vi "ST_parse_reference_list.vi"(6 "recordset_data":variant[][](array[variant]), 8 "error_in":errorcluster, 11 "command_nmb":u8) -> (0 "error_out":errorcluster, 3 "reference_data_to_PLC":u8[](array[numeric]))   [LabVIEW 2020]
uses:
  ST_reference_info.ctl
  _misc/byte_array_parser/from_STR_to_PLC_STRING[30].vi
  reference_byte_offsset/ref_STRING_offset.vi
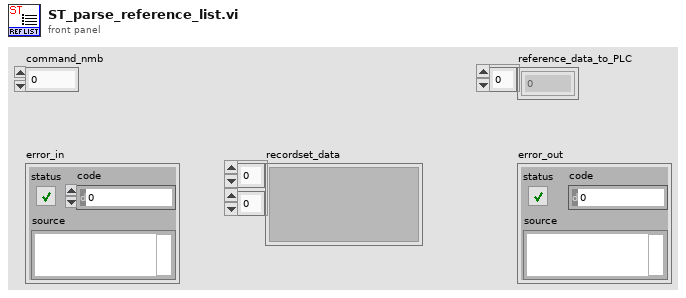
[diagram p1: front panel]
types:
  T1 = typedef "ST_reference_info.ctl" = cluster{"INT_number":i32, "REAL_number":i32, "STRING_number":i32, "STRING_size":i32, "BYTE_array":u8[]}
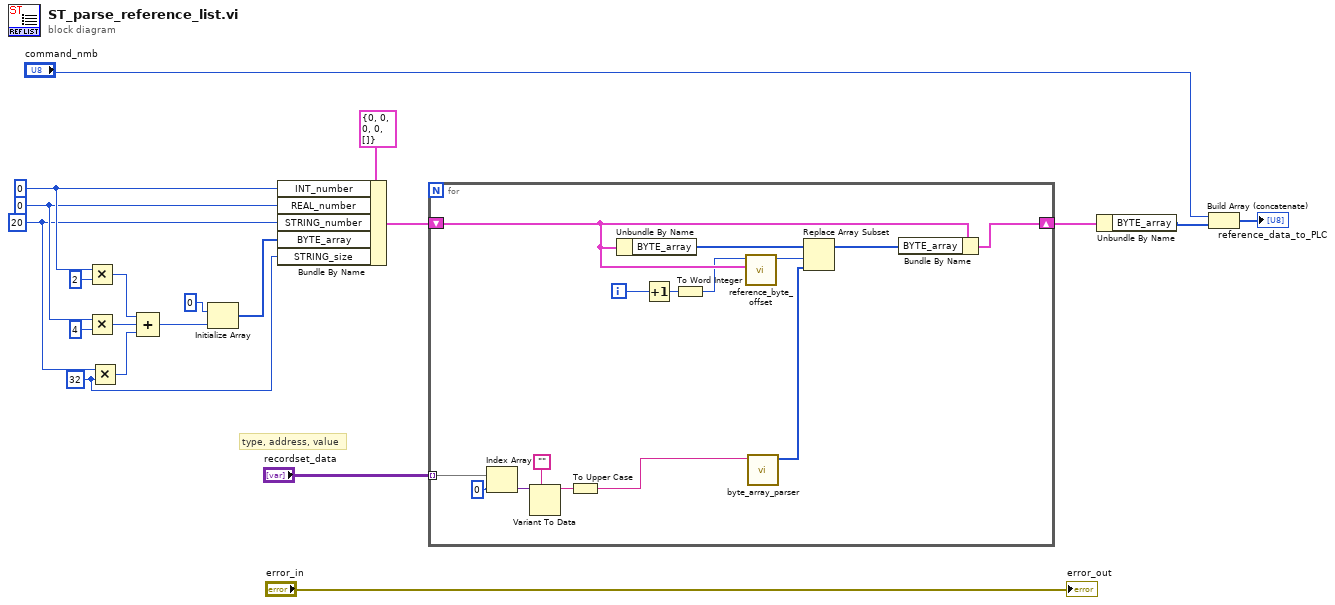
[diagram p0: block diagram]
diagram:
  w4 = 32 ("y")
  w5 = 20 ("STRING_number")
  w6 = 0 ("REAL_number")
  w7 = 0 ("INT_number")
  # "type, address, value"
  n1 = Multiply(x=w7, y=2) -> (x*y=w12:i32)
  n2 = Multiply(x=w6, y=4) -> (x*y=w11:i32)
  n3 = Multiply(x=w5, y=w4) -> (x*y=w10:i32)
  n4 = Compound Arithmetic op=unknown(w12, w11, w10) -> (w9:i32)
  n5 = Initialize Array(u8 0 ("element"), w9) -> (w15:u8[])
  n6 = Bundle By Name(cluster=T1 {"INT_number"=0, "REAL_number"=0, "STRING_number"=0, "STRING_size"=0, "BYTE_array"=[]}, "INT_number"=w7, "REAL_number"=w6, "STRING_number"=w5, "BYTE_array"=w15, "STRING_size"=w4) -> (w17:T1)
  n7 = for {
    tunnel: "recordset_data" -> [w30] mode=indexing
    shift-right: [w29] -> w8
    shift-left: w17 -> [w35]
    i -> [w23]
    n8 = Index Array(array=w30, index=0) -> (element=w33:variant)
    n9 = Variant To Data(type="", Variant=w33) -> (data=w31:string)  [unwired: 1 in, 1 out]
    n10 = To Upper Case(1:w31) -> (0:w24:string)
    n11 = Unbundle By Name(w35) -> ("BYTE_array"=w28:u8[])
    n12 = Increment(x=w23) -> (x+1=w22:i32)
    n13 = To Word Integer(number=w22) -> (16bit integer=w21:i16)
    n14 = call-poly "reference_byte_offset.vi"("ST_reference_info"=w35, "STRING_position"=w21) -> ("reference_byte_array_offset"=w25:i32)  [unwired: 9 in]
    n15 = call-poly "byte_array_parser.vi"("String"=w24) -> ("byte_array"=w26:u8[])  [unwired: 9 in, 1 out]
    n16 = Replace Array Subset(array=w28, new element=w26, index=w25) -> (w27:u8[])
    n17 = Bundle By Name(cluster=w35, "BYTE_array"=w27) -> (w29:T1)
  }
  n18 = Unbundle By Name(w8) -> ("BYTE_array"=w3:u8[])
  n19 = Build Array (concatenate)("command_nmb", w3) -> (→"reference_data_to_PLC":u8[])
  "error_out" <- "error_in"
